vi "Find Object Item Offset by Name.vi"(7 "Item Name <JSON>":string, 10 "Object Offset":i32, 11 "JSON":string) -> (0 "Found":bool, 1 "Offset past Item (or past last Item, if not found)":i32, 2 "Item Offset (-1 if not found)":i32, 3 "State":T1, 4 "Empty Object":bool)   [LabVIEW 2019, in "JSONtext.lvlib"]
uses:
  JSONtext.lvlib
  Parsing/Parsing State.ctl
  Parsing/Advance past Line Ending.vi
  Parsing/Advance past String.vi
  Parsing/Advance past Number.vi
  Parsing/Advance past Array.vi
  Parsing/Advance past Object.vi
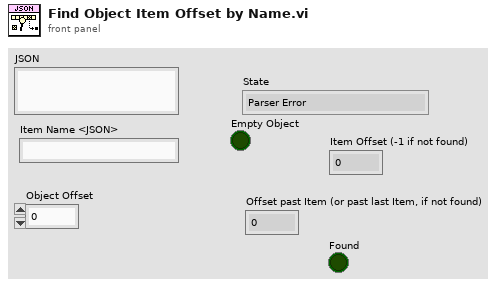
[diagram p1: front panel]
types:
  T1 = typedef "JSONtext.lvlib/Parsing State.ctl" = enum16{"Parser Error", "Object", "Array", "String", "Number/Other", "Leading Whitespace", "Object end", "Array end", "Value end"}
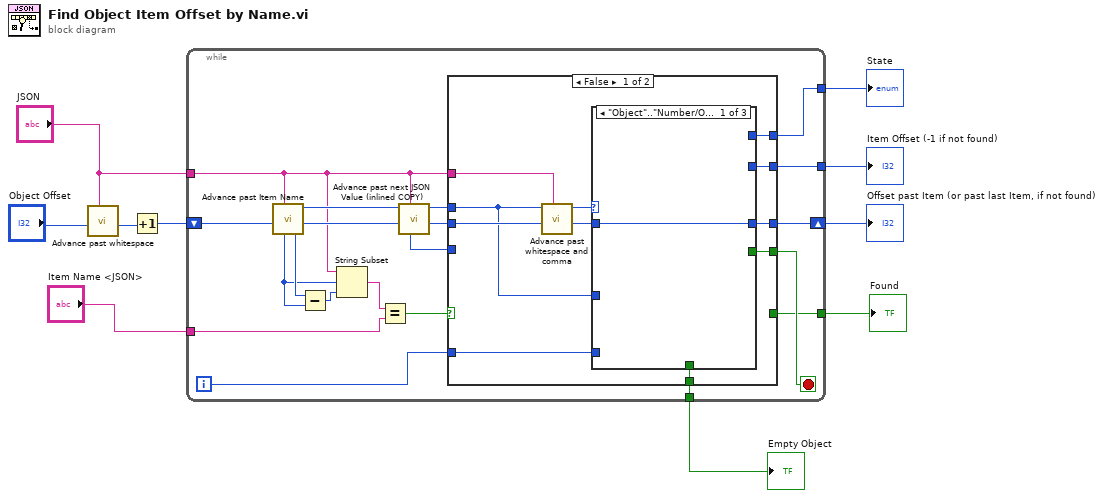
[diagram p0: block diagram]
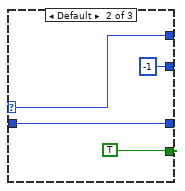
[diagram p2: hidden frame]
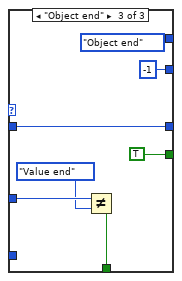
[diagram p3: hidden frame]
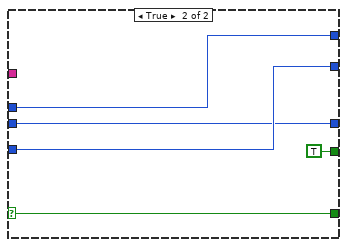
[diagram p4: hidden frame]
diagram:
  n1 = call "Advance past whitespace.vi"("JSON"="JSON", "Offset"="Object Offset") -> ("Offset of first non-whitespace"=w4:i32)  [unwired: 7 in, 2 out]
  n2 = Increment(x=w4) -> (x+1=w8:i32)
  n3 = while {
    shift-right: [w30] -> w9
    shift-left: w8 -> [w27]
    tunnel: "JSON" -> [w22]
    tunnel: [w28] -> w10
    tunnel: "Item Name <JSON>" -> [w19]
    tunnel: [w17] -> w6
    tunnel: [w16] -> w5
    tunnel: [w12] -> w1
    i -> [w13]
    stop <- w29 stop-if-true
    n4 = call "Advance past Item Name.vi"("JSON"=w22, "Offset"=w27) -> ("Offset past colon"=w24:i32, "State"=w25:T1, "Offset past Name"=w15:i32, "Name start out"=w14:i32)  [unwired: 6 in]
    n5 = Subtract(x=w15, y=w14) -> (x-y=w21:i32)
    n6 = String Subset(string=w22, offset (0)=w14, length (rest)=w21) -> (substring=w20:string)
    n7 = Equal?(x=w20, y=w19) -> (x = y?=w18:bool)
    n8 = call "Advance past next JSON Value (inlined COPY).vi"("JSON"=w22, "Offset"=w24, "State"=w25) -> ("Offset"=w23:i32, "State"=w26:T1, "Value start"=w11:i32)  [unwired: 4 in, 2 out]
    n9 = case shown="False" w18 {
      selector: w18 -> [_ w54]
      tunnel: [w40 w56] -> w30
      tunnel: [w39 TRUE] -> w29
      tunnel: [w38 w58] -> w28
      tunnel: w26 -> [w32 w58]
      tunnel: w23 -> [w36 w56]
      tunnel: w22 -> [w37 _]
      tunnel: w11 -> [_ w57]
      tunnel: [w34 w57] -> w17
      tunnel: [_ w54] -> w16
      tunnel: w13 -> [w33 _]
      tunnel: [w31 _] -> w12
      frame False {
        n10 = call "Advance past whitespace and comma.vi"("JSON"=w37, "Offset"=w36, "State in"=w32) -> ("Offset past match"=w35:i32, "State"=w41:T1)  [unwired: 6 in, 1 out]
        n11 = case shown="\"Object\"..\"Number/Other\"" w41 {
          selector: w41 -> [_ w43 _]
          tunnel: [_ TRUE TRUE] -> w39
          tunnel: [_ w43 Parsing_State."Object end"] -> w38
          tunnel: w35 -> [w42 w45 w50]
          tunnel: [w42 w45 w50] -> w40
          tunnel: [_ -1 -1] -> w34
          tunnel: w33 -> [_ _ _]
          tunnel: w32 -> [_ _ w49]
          tunnel: [_ _ w47] -> w31
          frame "Object".."Number/Other" {
          }
          frame Default {
          }
          frame "Object end" {
            n12 = Not Equal?(x=w49, y=Parsing_State."Value end") -> (x != y?=w47:bool)
          }
        }
      }
      frame True {
      }
    }
  }
  "State" <- w10
  "Offset past Item (or past last Item, if not found)" <- w9
  "Item Offset (-1 if not found)" <- w6
  "Found" <- w5
  "Empty Object" <- w1
